vi "ReportedTempWithinTolerance.vi"(1 "Temp Tolerance (C)":dbl=1.5 min=0.0 max=5.0 step=0.01 format="%0.2f", 2 "Set Temp (C)":dbl, 3 "Reported Temp (C)":dbl) -> (0 "Pass":bool)   [LabVIEW 2012]
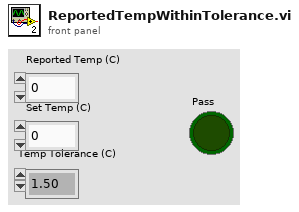
[diagram p1: front panel]
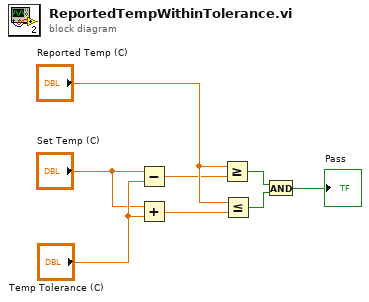
[diagram p0: block diagram]
diagram:
  n1 = Subtract(x="Set Temp (C)", y="Temp Tolerance (C)") -> (x-y=w2:dbl)
  n2 = Add(x="Set Temp (C)", y="Temp Tolerance (C)") -> (x+y=w1:dbl)
  n3 = Greater Or Equal?(x="Reported Temp (C)", y=w2) -> (x >= y?=w7:bool)
  n4 = Less Or Equal?(x="Reported Temp (C)", y=w1) -> (x <= y?=w6:bool)
  n5 = And(x=w7, y=w6) -> (x .and. y?=→"Pass":bool)
